vi "Smoothing Filter Coefficients.vi"(6 "fs":dbl=0.01 format="%0.2f", 8 "time constant":dbl=0.1 format="%.2f", 9 "shape":enum16{"rectangular", "triangular"}(ring), 10 "half-width":i32=1, 11 "type":enum16{"moving average", "exponential"}(ring)) -> (0 "error":i32, 2 "forward coefficients":dbl[](array[numeric]), 3 "reverse coefficients":dbl[](array[numeric]))   [LabVIEW 2024, in "NI_AALBase.lvlib"]
doc: "<p>Designs filter coefficients for a smoothing filter. You can use this VI to design a moving-average FIR filter or an exponentially-averaging IIR filter.</p>"
uses:
  NI_AALBase.lvlib
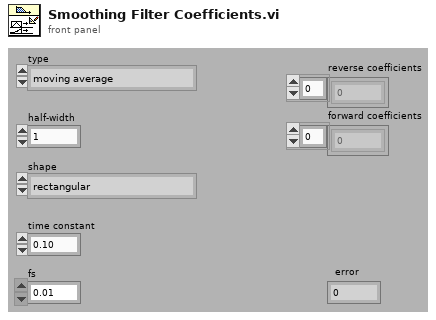
[diagram p1: front panel]
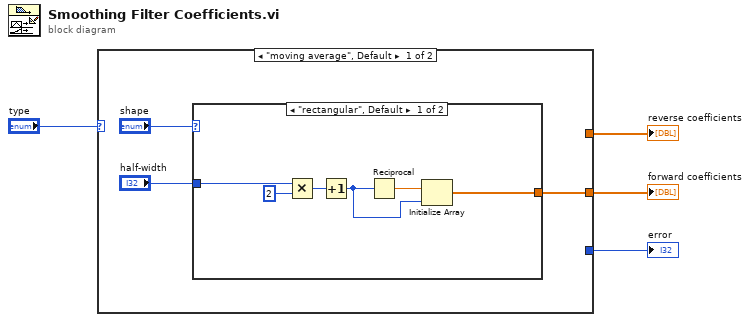
[diagram p0: block diagram]
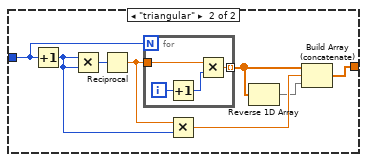
[diagram p2: hidden frame]
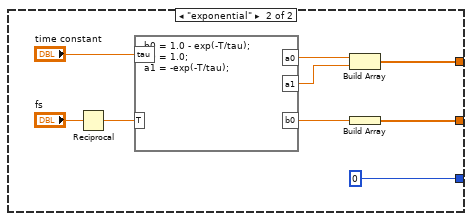
[diagram p3: hidden frame]
diagram:
  n1 = case shown="\"moving average\", Default" "type" {
    tunnel: [w6 w33] -> w3
    tunnel: [_ w34] -> w2
    tunnel: [_ 0 ("error")] -> w1
    frame "moving average", Default {
      n2 = case shown="\"rectangular\", Default" "shape" {
        tunnel: [w12 w15] -> w6
        tunnel: "half-width" -> [w9 w14]
        frame "rectangular", Default {
          n3 = Multiply(x=w9, y=2 ("x")) -> (x*y=w10:i32)
          n4 = Increment(x=w10) -> (x+1=w8:i32)
          n5 = Reciprocal(x=w8) -> (1/x=w13:dbl)
          n6 = Initialize Array(w13, w8) -> (w12:dbl[])
        }
        frame "triangular" {
          n7 = Increment(x=w14) -> (x+1=w19:i32)
          n8 = Multiply(x=w19, y=w19) -> (x*y=w21:i32)
          n9 = Reciprocal(x=w21) -> (1/x=w20:dbl)
          n10 = for {
            N: w14 -> [_]
            tunnel: w20 -> [w24]
            tunnel: [w23] -> w17 mode=indexing
            i -> [w25]
            n11 = Increment(x=w25) -> (x+1=w22:i32)
            n12 = Multiply(x=w24, y=w22) -> (x*y=w23:dbl)
          }
          n13 = Multiply(x=w20, y=w19) -> (x*y=w18:dbl)
          n14 = Reverse 1D Array(array=w17) -> (reversed array=w16:dbl[])
          n15 = Build Array (concatenate)(w17, w18, w16) -> (w15:dbl[])
        }
      }
    }
    frame "exponential" {
      n16 = Reciprocal(x="fs") -> (1/x=w27:dbl)
      n17 = formula code="b0 = 1.0 - exp(-T/tau);\na0 = 1.0;\na1 = -exp(-T/tau);"("tau"="time constant", "T"=w27) -> ("b0"=w30:dbl, "a0"=w29:dbl, "a1"=w28:dbl)
      n18 = Build Array(w29, w28) -> (w34:dbl[])
      n19 = Build Array(w30) -> (w33:dbl[])
    }
  }
  "reverse coefficients" <- w2
  "forward coefficients" <- w3
  "error" <- w1
